vi "Been Called.vi"(8 "error in (no error)":errorcluster, 11 "LabSpy in":refnum<class "LabSpy.lvclass">) -> (0 "error out":errorcluster, 2 "Been Called":bool, 3 "LabSpy out":refnum<class "LabSpy.lvclass">)   [LabVIEW 2013, in "LabSpy.lvclass"]
uses:
  LabSpy.lvclass
  LabSpy.lvclass/LabSpy.ctl
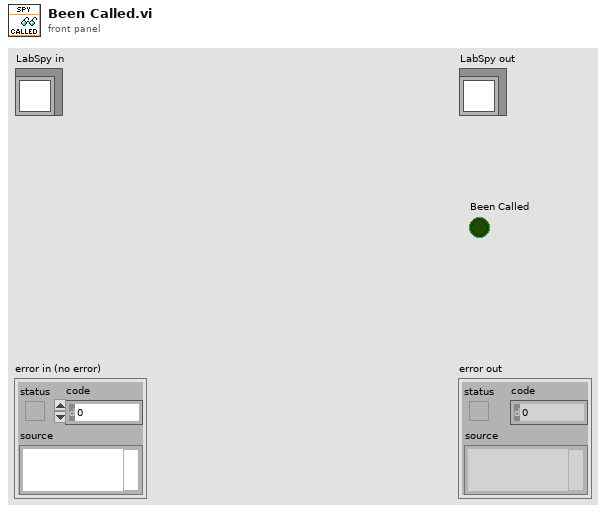
[diagram p1: front panel]
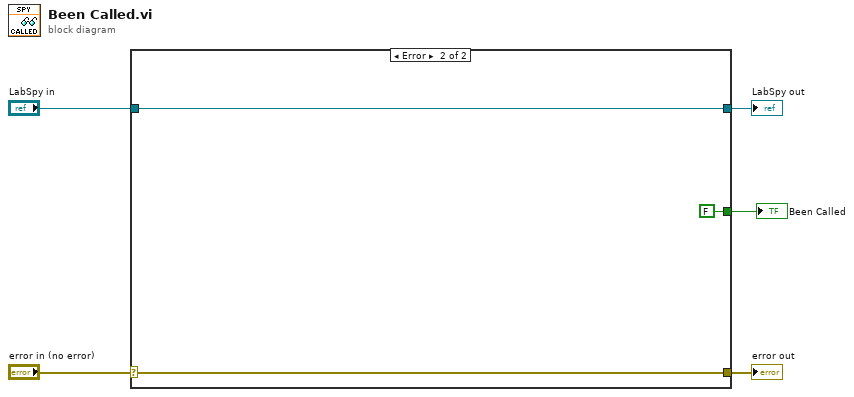
[diagram p0: block diagram]
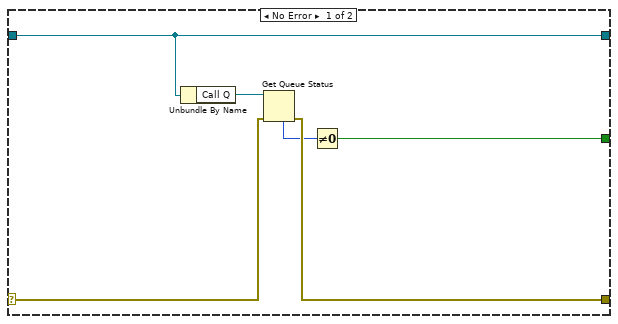
[diagram p2: hidden frame]
diagram:
  n1 = case shown="Error" "error in (no error)" {
    selector: "error in (no error)" -> [w9 w14]
    tunnel: [w8 w14] -> w4
    tunnel: [w11 w13] -> w2
    tunnel: "LabSpy in" -> [w11 w13]
    tunnel: [w6 FALSE] -> w1
    frame No Error {
      n2 = Unbundle By Name(w11) -> ("Call Q"=w10:refnum<queue>)
      n3 = Get Queue Status(queue=w10, error in (no error)=w9) -> (error out=w8:errorcluster, # elements in queue=w7:i32)  [unwired: 1 in, 6 out]
      n4 = Not Equal To 0?(x=w7) -> (x != 0?=w6:bool)
    }
    frame Error {
    }
  }
  "error out" <- w4
  "LabSpy out" <- w2
  "Been Called" <- w1
